vi "main.vi"() -> ()   [LabVIEW 2021]
panel:
  out "error out 2":errorcluster
  out "error out":errorcluster
  in  "vi path":path=path "D:/git/LabVIEW/ui-automation/labview-ui-testing/Prototype/ExeSubPanel - Copy/VI 2.vi"
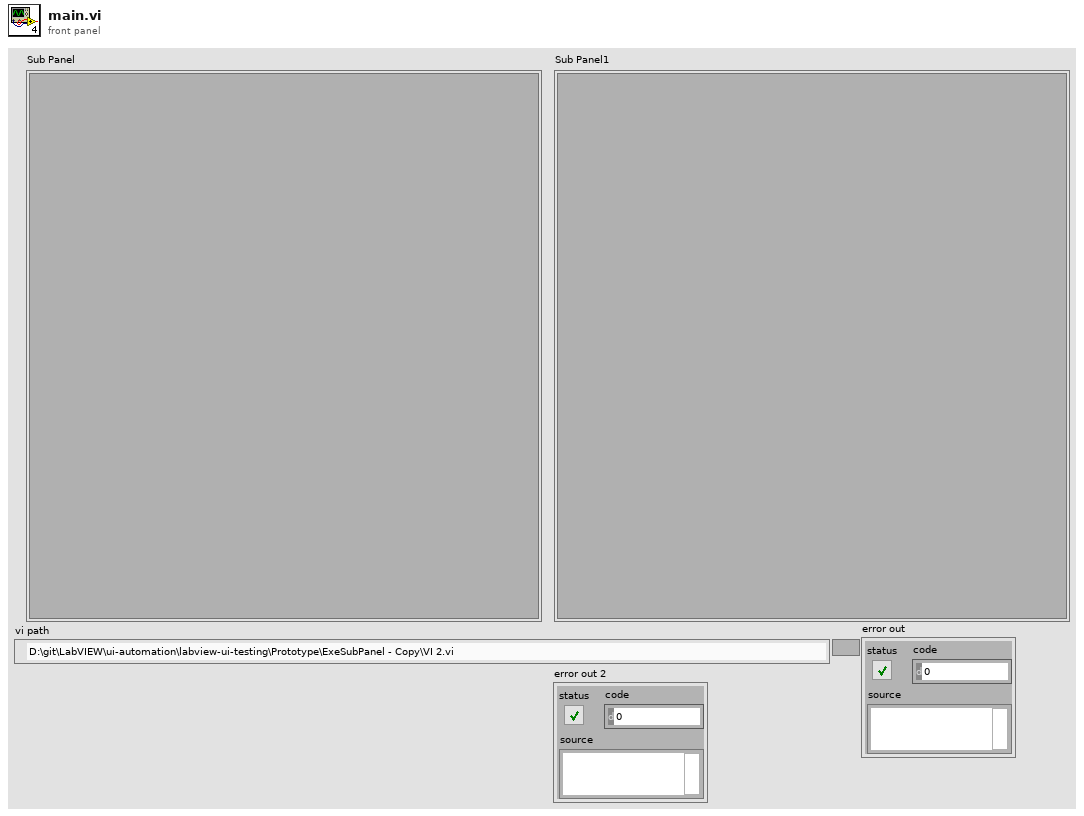
[diagram p1: front panel]
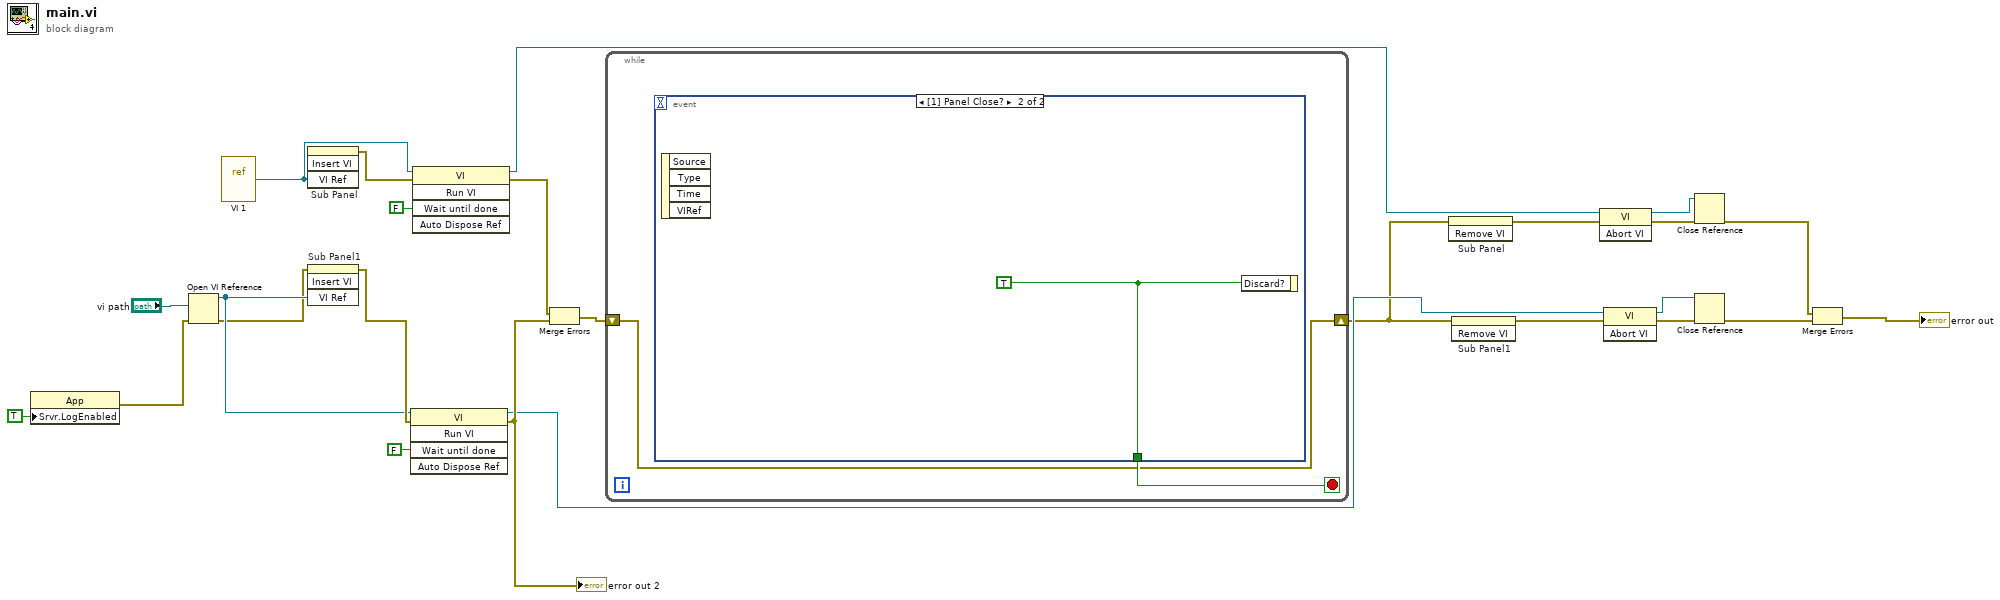
[diagram p0: block diagram]
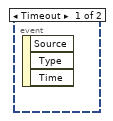
[diagram p2: hidden frame]
diagram:
  n1 = property class="App"("Srvr.LogEnabled"=TRUE ("Server:Logging Enabled")) -> (error out=w2:errorcluster)  [unwired: 2 in, 1 out]
  n2 = Open VI Reference(vi path="vi path", error in (no error)=w2) -> (vi reference=w20:refnum<vi>, error out=w19:errorcluster)  [unwired: 4 in]
  n3 = vi-ref "VI 1.vi"() -> (w25:refnum<vi>)
  n4 = invoke on="Sub Panel" class="SubPnl" method="Insert VI"("VI Ref"=w25) -> (error out=w24:errorcluster)  [unwired: 3 in, 3 out]
  n5 = invoke on="Sub Panel1" class="SubPnl" method="Insert VI"(error in=w19, "VI Ref"=w20) -> (error out=w22:errorcluster)  [unwired: 2 in, 3 out]
  n6 = invoke class="VI" method="Run VI"(reference=w20, error in=w22, "Wait until done"=FALSE ("Wait Until Done")) -> (reference out=w12:refnum<vi>, error out=w21:errorcluster)  [unwired: 2 in, 3 out]
  "error out 2" <- w21
  n7 = invoke class="VI" method="Run VI"(reference=w25, error in=w24, "Wait until done"=FALSE ("Wait Until Done")) -> (reference out=w10:refnum<vi>, error out=w16:errorcluster)  [unwired: 2 in, 3 out]
  n8 = Merge Errors(w16, w21) -> (w17:errorcluster)
  n9 = while {
    shift-right: [w26] -> w4
    shift-left: w17 -> [w26]
    stop <- w27 stop-if-true
    n10 = event shown="[1] Panel Close?" {
      selector: _ -> [_ _]
      dyn-events: _ -> [_ _]
      timeout: _ -> [_ _]
      tunnel: [_ w28] -> w27
      event Timeout {
        n11 = event-data() -> ()  [unwired: 1 in, 3 out]
      }
      event Panel Close? {
        w28 = TRUE ("Discard?")
        n12 = event-data() -> ()  [unwired: 1 in, 4 out]
        n13 = event-data("Discard?"=w28) -> ()  [unwired: 1 in, 1 out]
      }
    }
  }
  n14 = invoke on="Sub Panel" class="SubPnl" method="Remove VI"(error in=w4) -> (error out=w5:errorcluster)  [unwired: 2 in, 2 out]
  n15 = invoke on="Sub Panel1" class="SubPnl" method="Remove VI"(error in=w4) -> (error out=w3:errorcluster)  [unwired: 2 in, 2 out]
  n16 = invoke class="VI" method="Abort VI"(reference=w10, error in=w5) -> (reference out=w8:refnum<vi>, error out=w9:errorcluster)  [unwired: 1 in, 1 out]
  n17 = invoke class="VI" method="Abort VI"(reference=w12, error in=w3) -> (reference out=w11:refnum<vi>, error out=w13:errorcluster)  [unwired: 1 in, 1 out]
  n18 = Close Reference(reference=w8, error in (no error)=w9) -> (error out=w6:errorcluster)
  n19 = Close Reference(reference=w11, error in (no error)=w13) -> (error out=w18:errorcluster)
  n20 = Merge Errors(w6, w18) -> (→"error out":errorcluster)
